vi "Draw Description.vi"(0 "DNL_Image In":picture, 1 "DNL_Documentation Path":path, 3 "DNL_Link color":u32(colorbox), 5 "DNL_String":string="Jump to the jam, boogie woogie jam slam.  Bust a dialect, I'm the man with the plan.  Come flow with the sounds of the mighty mic master, rhymin' on the microphone, and suckas, a disaster!", 7 "Underline Link?":bool caption="下划线链接？", 9 "DNL_Word Wrap Bound":u32=180, 11 "DNL_Text color":u32(colorbox), 13 "DNL_Point":T1={"Horizontal"=-1, "Vertical"=-1}, 14 "DNL_BG color":u32(colorbox)) -> (4 "DNL_Image Out":picture, 6 "End of Desc Character":i32 caption="说明信息结束字符", 8 "Hovering Over Link?":bool caption="悬停链接？")   [LabVIEW 2016, in "MetaDataObj.lvclass"]
uses:
  <resource>/dialog/NewProjectWizard/MetaDataObj/MetaDataObj.lvclass
  <vilib>/Utility/miscctls.llb/LVPoint32TypeDef.ctl
panel:
  in  "Project Information":string="更多信息" caption="项目信息"
  in  "DNL_#lines":u8=2
  in  "DNL_DisplayString":string
  # "请勿移动该控件...该控件因故位于前面板的原点处。"
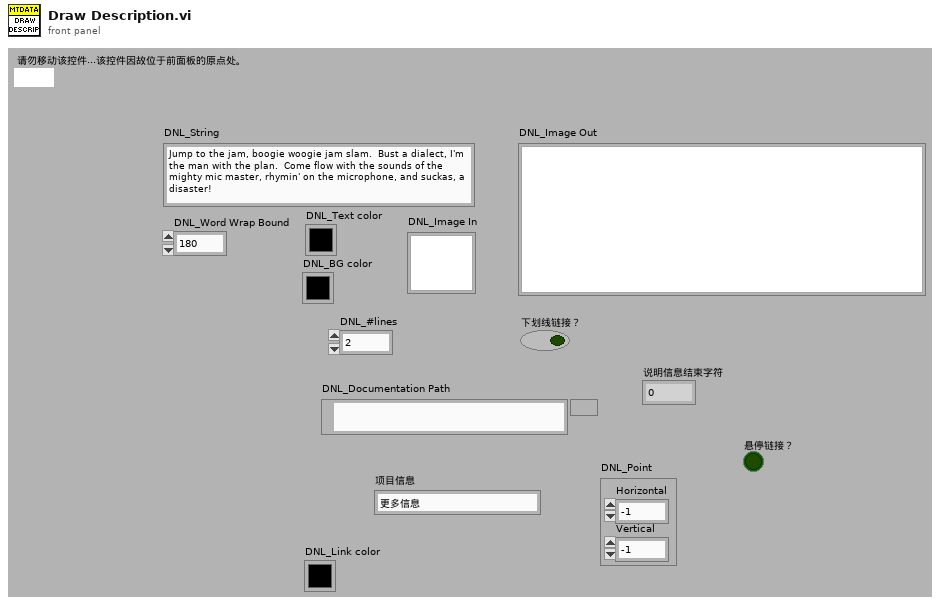
[diagram p1: front panel]
types:
  T1 = typedef "LVPoint32TypeDef.ctl" = cluster{"Horizontal":i32, "Vertical":i32}
  T2 = enum32{"invalid OS target", "Mac OS", "Windows 3.1", "Windows 95/NT", "Solaris 1", "Solaris 2", "HP-UX", "PowerMAX", "Linux", "Irix", "Rhapsody", "BeOS", "AIX", "OSF1", "VxWorks", "PharLap", "Carbon", "RTX", "Windows x64", "Linux x64"}
  T3 = enum32{"invalid OS target", "Mac OS", "Windows 3.1", "Windows 95/NT", "Solaris 1", "Solaris 2", "HP-UX", "PowerMAX", "Linux", "Irix", "Rhapsody", "BeOS", "AIX", "OSF1", "VxWorks", "PharLap", "Carbon", "RTX", "Windows x64", "Linux x64", "Mac OS X x64"}
  T4 = typedef "imagedata.ctl" = cluster{"image type":i32, "image depth":i32, "image":u8[], "mask":u8[], "colors":u32[], "Rectangle":cluster{"left":i16, "top":i16, "right":i16, "bottom":i16}}
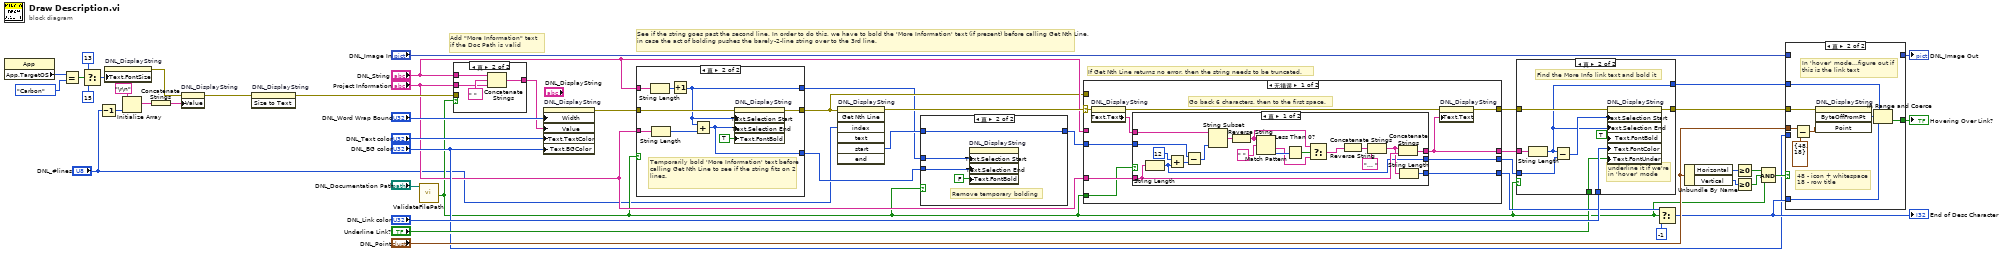
[diagram p0: block diagram]
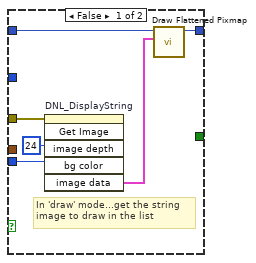
[diagram p4: hidden frame]
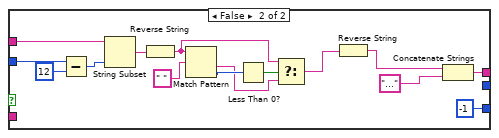
[diagram p7: hidden frame]
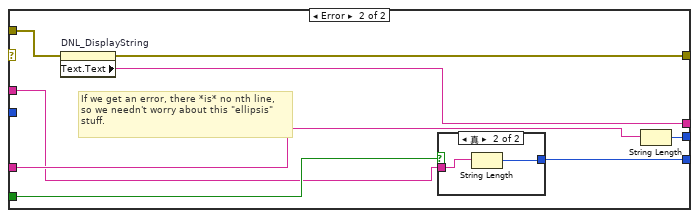
[diagram p8: hidden frame]
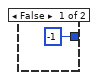
[diagram p9: hidden frame]
diagram:
  # "If Get Nth Line returns no error, then the string needs to be truncated."
  # "See if the string goes past the second line. In order to do this, we have to bold the 'More Information' text (if present) before calling Get Nth Line, in case the act of bolding pushes the barely-2-line string over to the 3rd line."
  # "Add \"More Information\" text\nif the Doc Path is valid"
  n1 = property class="App"() -> ("App.TargetOS"=w17:T3)  [unwired: 2 in, 2 out]
  n2 = Equal?(x=w17, y=T2."Carbon") -> (x = y?=w15:bool)
  n3 = Select(t=u32 13 ("Text.Font:Size"), s=w15, f=u32 15 ("Text.Font:Size")) -> (s? t:f=w11:u32)
  n4 = Decrement(x="DNL_#lines") -> (x-1=w18:u8)
  n5 = property on="DNL_DisplayString" class="Str"("Text.FontSize"=w11) -> (error out=w14:errorcluster)  [unwired: 2 in, 1 out]
  n6 = Initialize Array("\r\n", w18) -> (w22:string[])
  n7 = Concatenate Strings(w22) -> (w21:string)
  n8 = property on="DNL_DisplayString" class="Str"(error in=w14, "Value"=w21) -> (error out=w20:errorcluster)  [unwired: 1 in, 1 out]
  n9 = invoke on="DNL_DisplayString" class="Str" method="Size to Text"(error in=w20) -> (error out=w19:errorcluster)  [unwired: 2 in, 2 out]
  n10 = call <resource>:"ValidateFilePath.vi"("File Path In"="DNL_Documentation Path") -> ("Valid File Path?"=w6:bool)  [unwired: 9 in, 1 out]
  n11 = case shown="真" w6 {
    tunnel: "DNL_String" -> [w49 w53]
    tunnel: [w49 w52] -> w37
    tunnel: "Project Information" -> [_ w50]
    tunnel: w19 -> [_ _]
    frame False {
    }
    frame True {
      n12 = Concatenate Strings(w53, " ", w50) -> (w52:string)
    }
  }
  n13 = property on="DNL_DisplayString" class="Str"("Width"="DNL_Word Wrap Bound", "Value"=w37, "Text.TextColor"="DNL_Text color", "Text.BGColor"="DNL_BG color") -> (error out=w10:errorcluster)  [unwired: 2 in, 1 out]
  n14 = case shown="真" w6 {
    tunnel: w10 -> [w54 w59]
    tunnel: [w54 w58] -> w8
    tunnel: "DNL_String" -> [_ w63]
    tunnel: "Project Information" -> [_ w61]
    tunnel: [_ w56] -> w3
    tunnel: [_ w55] -> w2
    frame False {
    }
    frame True {
      # "Temporarily bold 'More Information' text before calling Get Nth Line to see if the string fits on 2 lines."
      n15 = String Length(string=w63) -> (length=w62:i32)
      n16 = String Length(string=w61) -> (length=w60:i32)
      n17 = Increment(x=w62) -> (x+1=w56:i32)
      n18 = Add(x=w56, y=w60) -> (x+y=w55:i32)
      n19 = property on="DNL_DisplayString" class="Str"(error in=w59, "Text.Selection Start"=w56, "Text.Selection End"=w55, "Text.FontBold"=TRUE ("Text.Font:Bold")) -> (error out=w58:errorcluster)  [unwired: 1 in, 1 out]
    }
  }
  n20 = invoke on="DNL_DisplayString" class="Str" method="Get Nth Line"(error in=w8, "index"="DNL_#lines") -> (error out=w46:errorcluster, "start"=w4:u32)  [unwired: 5 in, 5 out]
  n21 = case shown="真" w6 {
    tunnel: [w64 w68] -> w5
    tunnel: w4 -> [w64 w68]
    tunnel: w3 -> [_ w67]
    tunnel: w2 -> [_ w66]
    frame False {
    }
    frame True {
      # "Remove temporary bolding"
      n22 = property on="DNL_DisplayString" class="Str"("Text.Selection Start"=w67, "Text.Selection End"=w66, "Text.FontBold"=FALSE ("Text.Font:Bold")) -> ()  [unwired: 2 in, 2 out]
    }
  }
  n23 = case shown="无错误" w46 {
    selector: w46 -> [w77 _]
    tunnel: w5 -> [w78 _]
    tunnel: [w72 w119] -> w44
    tunnel: "Project Information" -> [w74 w114]
    tunnel: w6 -> [w73 w116]
    tunnel: [w71 w118] -> w42
    tunnel: w8 -> [_ w120]
    tunnel: [w70 w117] -> w40
    tunnel: [w69 w115] -> w38
    tunnel: "DNL_String" -> [_ w113]
    frame No Error {
      # "Go back 6 characters, then to the first space."
      n24 = property on="DNL_DisplayString" class="Str"(error in=w77) -> (error out=w75:errorcluster, "Text.Text"=w76:string)  [unwired: 1 in, 1 out]
      n25 = case shown="真" w73 {
        tunnel: w78 -> [w97 w112]
        tunnel: w76 -> [w96 w110]
        tunnel: [w91 w107] -> w71
        tunnel: w74 -> [w90 _]
        tunnel: [w89 -1] -> w70
        tunnel: [w87 _] -> w69
        frame True {
          n26 = String Length(string=w90) -> (length=w87:i32)
          n27 = Add(x=u32 12 ("y"), y=w87) -> (x+y=w92:u32)
          n28 = Subtract(x=w97, y=w92) -> (x-y=w95:u32)
          n29 = String Subset(string=w96, length (rest)=w95) -> (substring=w85:string)  [unwired: 1 in]
          n30 = Reverse String(1:w85) -> (0:w81:string)
          n31 = Match Pattern(string=w81, regular expression=" ") -> (after substring=w79:string, offset past match=w83:i32)  [unwired: 1 in, 2 out]
          n32 = Less Than 0?(x=w83) -> (x < 0?=w82:bool)
          n33 = Select(t=w81, s=w82, f=w79) -> (s? t:f=w80:string)
          n34 = Reverse String(1:w80) -> (0:w84:string)
          n35 = Concatenate Strings(w84, "... ") -> (w88:string)
          n36 = Concatenate Strings(w88, w90) -> (w91:string)
          n37 = String Length(string=w88) -> (length=w89:i32)
        }
        frame False {
          n38 = Subtract(x=w112, y=u32 12) -> (x-y=w109:u32)
          n39 = String Subset(string=w110, length (rest)=w109) -> (substring=w105:string)  [unwired: 1 in]
          n40 = Reverse String(1:w105) -> (0:w99:string)
          n41 = Match Pattern(string=w99, regular expression=" ") -> (after substring=w100:string, offset past match=w101:i32)  [unwired: 1 in, 2 out]
          n42 = Less Than 0?(x=w101) -> (x < 0?=w102:bool)
          n43 = Select(t=w99, s=w102, f=w100) -> (s? t:f=w98:string)
          n44 = Reverse String(1:w98) -> (0:w103:string)
          n45 = Concatenate Strings(w103, "...") -> (w107:string)
        }
      }
      n46 = property on="DNL_DisplayString" class="Str"(error in=w75, "Text.Text"=w71) -> (error out=w72:errorcluster)  [unwired: 1 in, 1 out]
    }
    frame Error {
      # "If we get an error, there *is* no nth line,\nso we needn't worry about this \"ellipsis\"\nstuff."
      n47 = property on="DNL_DisplayString" class="Str"(error in=w120) -> (error out=w119:errorcluster, "Text.Text"=w118:string)  [unwired: 1 in, 1 out]
      n48 = case shown="真" w116 {
        tunnel: [-1 w123] -> w117
        tunnel: w113 -> [_ w122]
        frame False {
        }
        frame True {
          n49 = String Length(string=w122) -> (length=w123:i32)
        }
      }
      n50 = String Length(string=w114) -> (length=w115:i32)
    }
  }
  n51 = case shown="真" w6 {
    tunnel: w44 -> [w124 w133]
    tunnel: [w124 w132] -> w43
    tunnel: w38 -> [_ w129]
    tunnel: w42 -> [_ w130]
    tunnel: "DNL_Link color" -> [_ w127]
    tunnel: [_ w125] -> w28
    tunnel: "Underline Link?" -> [_ w126]
    frame False {
    }
    frame True {
      # "underline it if we're\nin 'hover' mode"
      # "Find the More Info link text and bold it"
      n52 = String Length(string=w130) -> (length=w125:i32)
      n53 = Subtract(x=w125, y=w129) -> (x-y=w128:i32)
      n54 = property on="DNL_DisplayString" class="Str"(error in=w133, "Text.Selection Start"=w128, "Text.Selection End"=w125, "Text.FontBold"=TRUE ("Text.Font:Bold"), "Text.FontColor"=w127, "Text.FontUnder"=w126) -> (error out=w132:errorcluster)  [unwired: 1 in, 1 out]
    }
  }
  n55 = Select(t=w40, s=w6, f=-1) -> (s? t:f=w30:i32)
  "End of Desc Character" <- w30
  n56 = Unbundle By Name("DNL_Point") -> ("Horizontal"=w35:i32, "Vertical"=w34:i32)
  n57 = Greater Or Equal To 0?(x=w35) -> (x >= 0?=w33:bool)
  n58 = Greater Or Equal To 0?(x=w34) -> (x >= 0?=w32:bool)
  n59 = Compound Arithmetic op=AND(w33, w32, w6) -> (w31:bool)
  n60 = case shown="真" w31 {
    tunnel: w43 -> [w135 w147]
    tunnel: "DNL_Point" -> [_ w146]
    tunnel: w30 -> [_ w142]
    tunnel: [_ w141] -> w29
    tunnel: w28 -> [_ w140]
    tunnel: "DNL_Image In" -> [w137 _]
    tunnel: [w136 _] -> w25
    tunnel: "DNL_BG color" -> [w134 _]
    frame False {
      # "In 'draw' mode...get the string\nimage to draw in the list"
      n61 = invoke on="DNL_DisplayString" class="Str" method="Get Image"(error in=w135, "image depth"=24 ("Image Depth"), "bg color"=w134) -> ("image data"=w138:T4)  [unwired: 3 in, 5 out]
      n62 = call <vilib>:"Draw Flattened Pixmap.vi"("image data"=w138, "picture"=w137) -> ("new picture"=w136:picture)  [unwired: 7 out]
    }
    frame True {
      # "48 - icon + whitespace\n18 - row title"
      # "In 'hover' mode...figure out if\nthis is the link text"
      n63 = Subtract(x=w146, y=T1 {"Horizontal"=48, "Vertical"=18}) -> (x-y=w144:T1)
      n64 = invoke on="DNL_DisplayString" class="Str" method="ByteOffFromPt"(error in=w147, "Point"=w144) -> ("ByteOffFromPt"=w143:i32)  [unwired: 2 in, 3 out]
      n65 = In Range and Coerce(upper limit=w140, x=w143, lower limit=w142) -> (In Range?=w141:bool)  [unwired: 1 out]
    }
  }
  "DNL_Image Out" <- w25
  "Hovering Over Link?" <- w29
